vi "drive_straight_camera.vi"(10 "Speed (ft/sec)":dbl, 11 "Distance":dbl) -> ()   [LabVIEW 2012]
uses:
  Robot Global Data.vi
  <vilib>/Rock Robotics/WPI/RobotDrive/WPI_RobotDriveMecanumDrive_Cartesian.vi
  <vilib>/Rock Robotics/WPI/RobotDrive/WPI_RobotDriveGetSetRefNum.vi
panel:
  # "Use Encoder to scale distance,"
  # "Speed setting +/- 1 Full Scale"
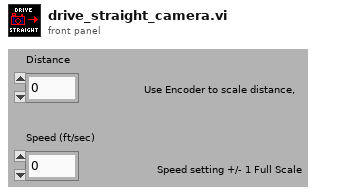
[diagram p1: front panel]
types:
  T1 = cluster{"Position":cluster{"X":dbl, "Y":dbl}, "Distance (ft)":dbl}[]
  T2 = cluster{"Position":cluster{"X":dbl, "Y":dbl}, "Distance (ft)":dbl}
  T3 = typedef "WPI_RobotDriveDevRef.ctl" = cluster{"DevStatus":errorcluster, "Motors[]":T4[], "Square Inputs":bool, "Max Output":dbl, "Isochronous":bool}
  T4 = typedef "WPI_MotorControlDeviceRef.ctl" = cluster{"DeviceStatus":errorcluster, "Type":enum16{"PWM", "CAN"}, "PWM":cluster{"Digital Module":T5, "PWM Channel":T6, "DeadBand":T7}, "CAN":cluster{"Device Number":u8, "Control Mode":T8, "Semaphore":T9, "Max Vout":dbl}, "Invert":bool, "TransformRef":T10, "InvTransformRef":T10}
  T5 = typedef "FPGA_TypedefDigitalModule.ctl" = enum16{"Digital Module 1", "Digital Module 2"}
  T6 = typedef "FPGA_DIOPWMChannel.ctl" = enum8{"PWM 1", "PWM 2", "PWM 3", "PWM 4", "PWM 5", "PWM 6", "PWM 7", "PWM 8", "PWM 9", "PWM 10", "Invalid"}
  T7 = typedef "WPI_PWMDeadband.ctl" = cluster{"Name":string, "maxPositivePwm":i32, "minPositivePwm":i32, "centerPwm":i32, "maxNegativePwm":i32, "minNegativePwm":i32, "angularRange":u16}
  T8 = typedef "WPI_CANJaguar_ControlMode.ctl" = enum8{"Percent VBus", "Current", "Speed", "Position", "Voltage"}
  T9 = typedef "Semaphore RefNum" = refnum<k1>
  T10 = typedef "WPI_PWMTransform_ConPane.ctl" = refnum<vi>
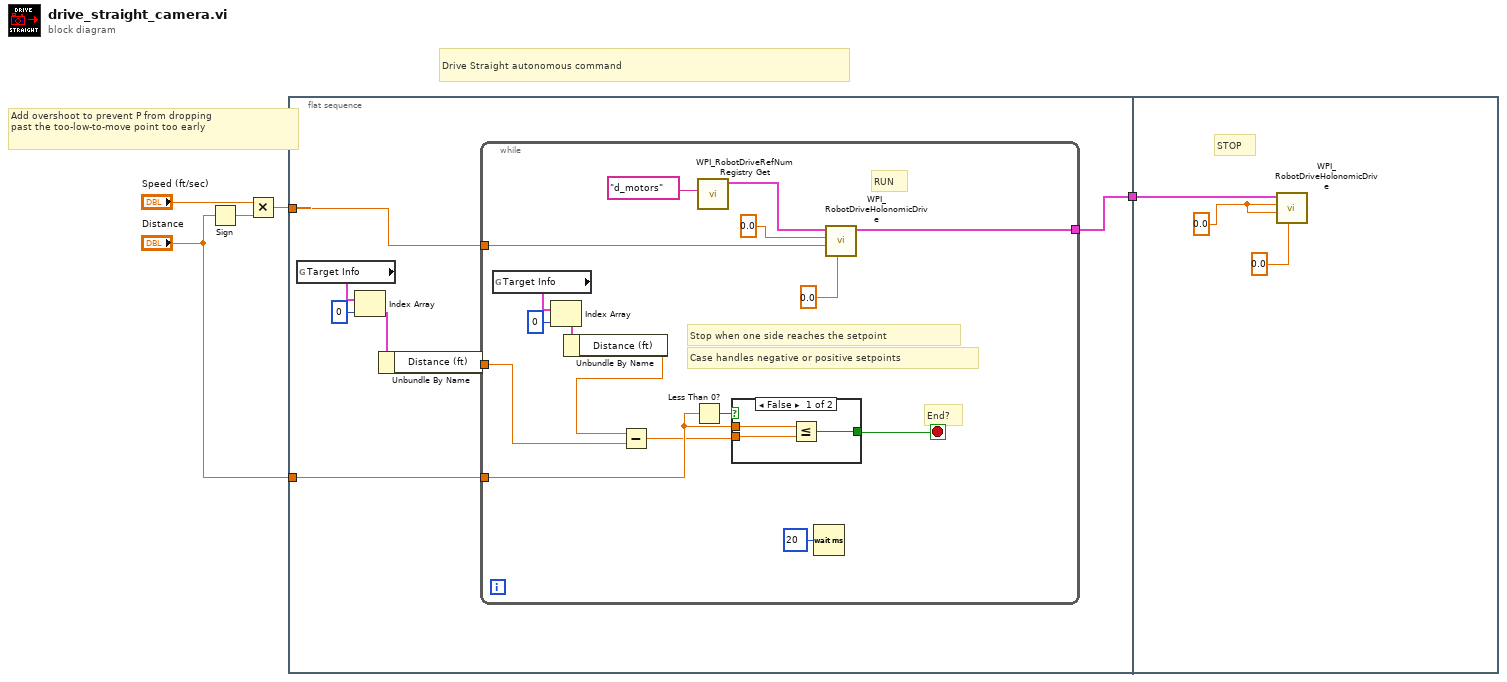
[diagram p0: block diagram]
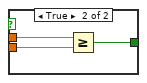
[diagram p2: hidden frame]
diagram:
  # "Drive Straight autonomous command"
  # "Add overshoot to prevent P from dropping\npast the too-low-to-move point too early"
  n1 = Sign(1:"Distance") -> (0:w3:dbl)
  n2 = Multiply(x="Speed (ft/sec)", y=w3) -> (x*y=w5:dbl)
  n3 = flat-sequence {
    tunnel: w5 -> [w12]
    tunnel: "Distance" -> [w11]
    tunnel: [w10] -> w1
    tunnel: w1 -> [w35]
    frame #0 {
      n4 = global read "Robot Global Data.vi" "Target Info"() -> (w8:T1)
      n5 = Index Array(array=w8, index=0) -> (element=w7:T2)
      n6 = Unbundle By Name(w7) -> ("Distance (ft)"=w6:dbl)
      n7 = while {
        tunnel: w12 -> [w23]
        tunnel: w6 -> [w25]
        tunnel: w11 -> [w26]
        tunnel: [w19] -> w10
        stop <- w13 stop-if-true
        # "RUN"
        # "Case handles negative or positive setpoints"
        # "End?"
        # "Stop when one side reaches the setpoint"
        n8 = global read "Robot Global Data.vi" "Target Info"() -> (w17:T1)
        n9 = Index Array(array=w17, index=0) -> (element=w18:T2)
        n10 = Unbundle By Name(w18) -> ("Distance (ft)"=w15:dbl)
        n11 = Subtract(x=w15, y=w25) -> (x-y=w14:dbl)
        n12 = Less Than 0?(x=w26) -> (x < 0?=w27:bool)
        n13 = call <vilib>:"WPI_RobotDriveRefNum Registry Get.vi"("refnum name"="d_motors") -> ("RobotDriveDevRef"=w22:T3)  [unwired: 1 in, 9 out]
        n14 = case shown="False" w27 {
          tunnel: w26 -> [w31 w34]
          tunnel: w14 -> [w30 w33]
          tunnel: [w29 w32] -> w13
          frame False {
            n15 = Less Or Equal?(x=w31, y=w30) -> (x <= y?=w29:bool)
          }
          frame True {
            n16 = Greater Or Equal?(x=w34, y=w33) -> (x >= y?=w32:bool)
          }
        }
        n17 = Wait (ms)(milliseconds to wait=u32 20) -> ()  [unwired: 1 out]
        n18 = call-poly <vilib>:"WPI_RobotDriveHolonomicDrive.vi"("Rotation"=0.0, "Y"=w23, "X"=0.0, "RobotDriveDevRef"=w22) -> ("RobotDriveDevRef"=w19:T3)  [unwired: 5 in, 2 out]
      }
    }
    frame #1 {
      w36 = 0.0 ("X")
      # "STOP"
      n19 = call-poly <vilib>:"WPI_RobotDriveHolonomicDrive.vi"("Rotation"=0.0, "Y"=w36, "X"=w36, "RobotDriveDevRef"=w35) -> ()  [unwired: 5 in, 3 out]
    }
  }
